vi "Project.vi"() -> ()   [LabVIEW 2016]
uses:
  <vilib>/DAQmx/read.llb/DAQmx Read (Digital Bool 1Line 1Point).vi
  <vilib>/DAQmx/write.llb/DAQmx Write (Digital Bool 1Line 1Point).vi
  <vilib>/DAQmx/create/channels.llb/DAQmx Create Channel (DI-Digital Input).vi
  <vilib>/DAQmx/create/channels.llb/DAQmx Create Channel (DO-Digital Output).vi
  <vilib>/DAQmx/miscellaneous.llb/DAQmx Fill In Error Info.vi
panel:
  in  "stop":bool
  out "Conveyor":bool
  out "STOP":bool
  out "START":bool
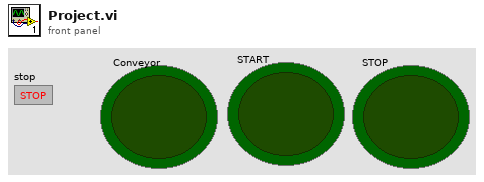
[diagram p1: front panel]
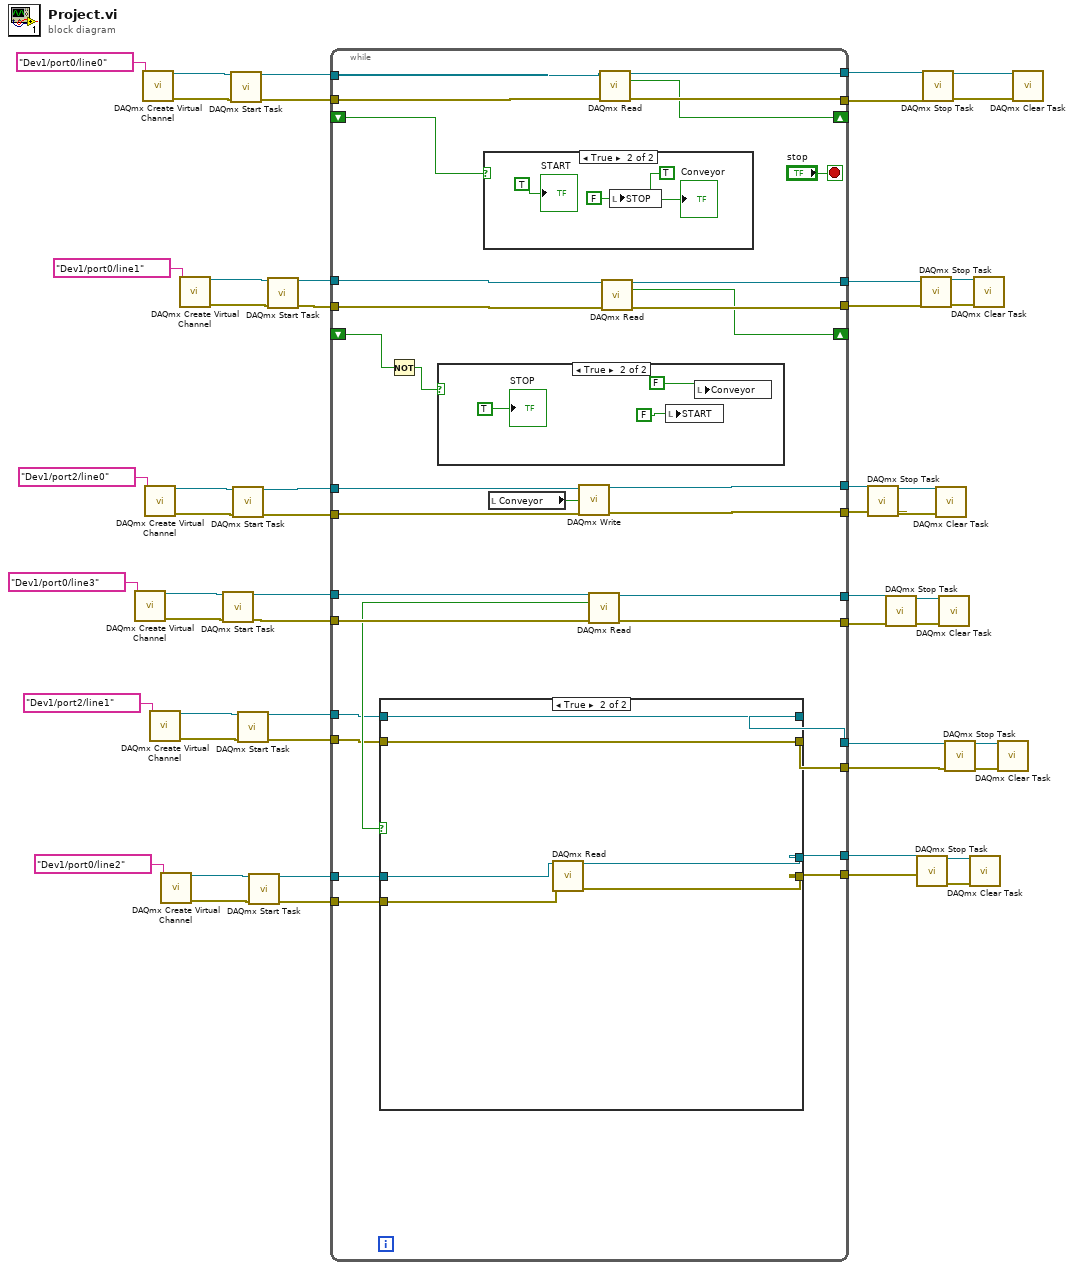
[diagram p0: block diagram]
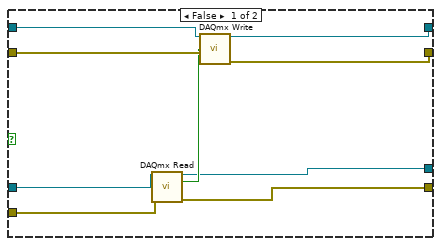
[diagram p2: hidden frame]
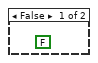
[diagram p3: hidden frame]
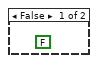
[diagram p4: hidden frame]
diagram:
  n1 = call-poly <vilib>:"DAQmx Create Virtual Channel.vi"("lines"=tag "Dev1/port0/line3") -> ("task out"=w27:refnum<k21>, "error out"=w26:errorcluster)  [unwired: 13 in]
  n2 = call-poly <vilib>:"DAQmx Create Virtual Channel.vi"("lines"=tag "Dev1/port0/line0") -> ("task out"=w54:refnum<k21>, "error out"=w53:errorcluster)  [unwired: 13 in]
  n3 = call-poly <vilib>:"DAQmx Create Virtual Channel.vi"("lines"=tag "Dev1/port2/line0") -> ("task out"=w38:refnum<k21>, "error out"=w37:errorcluster)  [unwired: 13 in]
  n4 = call-poly <vilib>:"DAQmx Create Virtual Channel.vi"("lines"=tag "Dev1/port2/line1") -> ("task out"=w14:refnum<k21>, "error out"=w13:errorcluster)  [unwired: 13 in]
  n5 = call-poly <vilib>:"DAQmx Create Virtual Channel.vi"("lines"=tag "Dev1/port0/line2") -> ("task out"=w5:refnum<k21>, "error out"=w4:errorcluster)  [unwired: 13 in]
  n6 = call-poly <vilib>:"DAQmx Create Virtual Channel.vi"("lines"=tag "Dev1/port0/line1") -> ("task out"=w46:refnum<k21>, "error out"=w45:errorcluster)  [unwired: 13 in]
  n7 = call <vilib>:"DAQmx Start Task.vi"("task/channels in"=w27, "error in"=w26) -> ("task out"=w24:refnum<k21>, "error out"=w23:errorcluster)  [unwired: 12 in]
  n8 = call <vilib>:"DAQmx Start Task.vi"("task/channels in"=w54, "error in"=w53) -> ("task out"=w52:refnum<k21>, "error out"=w51:errorcluster)  [unwired: 12 in]
  n9 = call <vilib>:"DAQmx Start Task.vi"("task/channels in"=w38, "error in"=w37) -> ("task out"=w36:refnum<k21>, "error out"=w35:errorcluster)  [unwired: 12 in]
  n10 = call <vilib>:"DAQmx Start Task.vi"("task/channels in"=w14, "error in"=w13) -> ("task out"=w11:refnum<k21>, "error out"=w10:errorcluster)  [unwired: 12 in]
  n11 = call <vilib>:"DAQmx Start Task.vi"("task/channels in"=w5, "error in"=w4) -> ("task out"=w2:refnum<k21>, "error out"=w1:errorcluster)  [unwired: 12 in]
  n12 = call <vilib>:"DAQmx Start Task.vi"("task/channels in"=w46, "error in"=w45) -> ("task out"=w42:refnum<k21>, "error out"=w41:errorcluster)  [unwired: 12 in]
  n13 = while {
    tunnel: w52 -> [w86]
    tunnel: w51 -> [w85]
    tunnel: [w84] -> w50
    tunnel: [w83] -> w49
    shift-right: [w82] -> _
    shift-left: _ -> [w81]
    tunnel: w42 -> [w80]
    tunnel: w41 -> [w79]
    tunnel: [w78] -> w40
    tunnel: [w77] -> w39
    shift-right: [w76] -> _
    shift-left: _ -> [w75]
    tunnel: w36 -> [w73]
    tunnel: w35 -> [w72]
    tunnel: [w71] -> w32
    tunnel: [w70] -> w31
    tunnel: w24 -> [w67]
    tunnel: w23 -> [w66]
    tunnel: [w65] -> w20
    tunnel: [w64] -> w19
    tunnel: [w60] -> w16
    tunnel: [w59] -> w15
    tunnel: w11 -> [w62]
    tunnel: w10 -> [w61]
    tunnel: [w58] -> w7
    tunnel: [w57] -> w6
    tunnel: w2 -> [w56]
    tunnel: w1 -> [w55]
    stop <- "stop" stop-if-true
    n14 = Not(x=w75) -> (.not. x?=w74:bool)
    n15 = case shown="True" w74 {
      frame False {
        (unwired) FALSE
      }
      frame True {
        n16 = local write "START"(FALSE) -> ()
        n17 = local write "Conveyor"(FALSE) -> ()
        "STOP" <- TRUE
      }
    }
    n18 = case shown="True" w81 {
      frame False {
        (unwired) FALSE
      }
      frame True {
        n19 = local write "STOP"(FALSE) -> ()
        "START" <- TRUE
        "Conveyor" <- TRUE
      }
    }
    n20 = local read "Conveyor"() -> (w68:bool)
    n21 = call-poly <vilib>:"DAQmx Write.vi"("task/channels in"=w73, "data"=w68, "error in"=w72) -> ("task out"=w71:refnum<k21>, "error out"=w70:errorcluster)  [unwired: 10 in, 1 out]
    n22 = call-poly <vilib>:"DAQmx Read.vi"("task/channels in"=w67, "error in"=w66) -> ("task out"=w65:refnum<k21>, "data"=w63:bool, "error out"=w64:errorcluster)  [unwired: 11 in]
    n23 = case shown="True" w63 {
      tunnel: w62 -> [w95 w101]
      tunnel: w61 -> [w94 w100]
      tunnel: [w93 w101] -> w60
      tunnel: [w92 w100] -> w59
      tunnel: [w90 w97] -> w58
      tunnel: [w89 w96] -> w57
      tunnel: w56 -> [w88 w99]
      tunnel: w55 -> [w87 w98]
      frame False {
        n24 = call-poly <vilib>:"DAQmx Read.vi"("task/channels in"=w88, "error in"=w87) -> ("task out"=w90:refnum<k21>, "data"=w91:bool, "error out"=w89:errorcluster)  [unwired: 11 in]
        n25 = call-poly <vilib>:"DAQmx Write.vi"("task/channels in"=w95, "data"=w91, "error in"=w94) -> ("task out"=w93:refnum<k21>, "error out"=w92:errorcluster)  [unwired: 10 in, 1 out]
      }
      frame True {
        n26 = call-poly <vilib>:"DAQmx Read.vi"("task/channels in"=w99, "error in"=w98) -> ("task out"=w97:refnum<k21>, "error out"=w96:errorcluster)  [unwired: 11 in, 1 out]
      }
    }
    n27 = call-poly <vilib>:"DAQmx Read.vi"("task/channels in"=w86, "error in"=w85) -> ("task out"=w84:refnum<k21>, "data"=w82:bool, "error out"=w83:errorcluster)  [unwired: 11 in]
    n28 = call-poly <vilib>:"DAQmx Read.vi"("task/channels in"=w80, "error in"=w79) -> ("task out"=w77:refnum<k21>, "data"=w76:bool, "error out"=w78:errorcluster)  [unwired: 11 in]
  }
  n29 = call <vilib>:"DAQmx Stop Task.vi"("task/channels in"=w32, "error in"=w31) -> ("task out"=w34:refnum<k21>, "error out"=w33:errorcluster)  [unwired: 12 in]
  n30 = call <vilib>:"DAQmx Stop Task.vi"("task/channels in"=w20, "error in"=w19) -> ("task out"=w22:refnum<k21>, "error out"=w21:errorcluster)  [unwired: 12 in]
  n31 = call <vilib>:"DAQmx Stop Task.vi"("task/channels in"=w7, "error in"=w6) -> ("task out"=w9:refnum<k21>, "error out"=w8:errorcluster)  [unwired: 12 in]
  n32 = call <vilib>:"DAQmx Stop Task.vi"("task/channels in"=w39, "error in"=w40) -> ("task out"=w44:refnum<k21>, "error out"=w43:errorcluster)  [unwired: 12 in]
  n33 = call <vilib>:"DAQmx Stop Task.vi"("task/channels in"=w50, "error in"=w49) -> ("task out"=w48:refnum<k21>, "error out"=w47:errorcluster)  [unwired: 12 in]
  n34 = call <vilib>:"DAQmx Clear Task.vi"("task in"=w34, "error in"=w33) -> ()  [unwired: 13 in, 1 out]
  n35 = call <vilib>:"DAQmx Clear Task.vi"("task in"=w22, "error in"=w21) -> ()  [unwired: 13 in, 1 out]
  n36 = call <vilib>:"DAQmx Stop Task.vi"("task/channels in"=w16, "error in"=w15) -> ("task out"=w18:refnum<k21>, "error out"=w17:errorcluster)  [unwired: 12 in]
  n37 = call <vilib>:"DAQmx Clear Task.vi"("task in"=w9, "error in"=w8) -> ()  [unwired: 13 in, 1 out]
  n38 = call <vilib>:"DAQmx Clear Task.vi"("task in"=w44, "error in"=w43) -> ()  [unwired: 13 in, 1 out]
  n39 = call <vilib>:"DAQmx Clear Task.vi"("task in"=w18, "error in"=w17) -> ()  [unwired: 13 in, 1 out]
  n40 = call <vilib>:"DAQmx Clear Task.vi"("task in"=w48, "error in"=w47) -> ()  [unwired: 13 in, 1 out]
